vi "dummy.vi"() -> ()   [LabVIEW 2021]
panel:
  in  "stop":bool
  in  "RPM":dbl(slide) scale=1.0..500.0
  out "Visualize":bool[](array[boolean])
  in  "Full Step":bool
  in  "Direction":enum32{"CW", "CCW"}(radio)
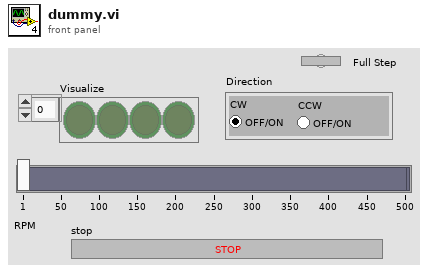
[diagram p1: front panel]
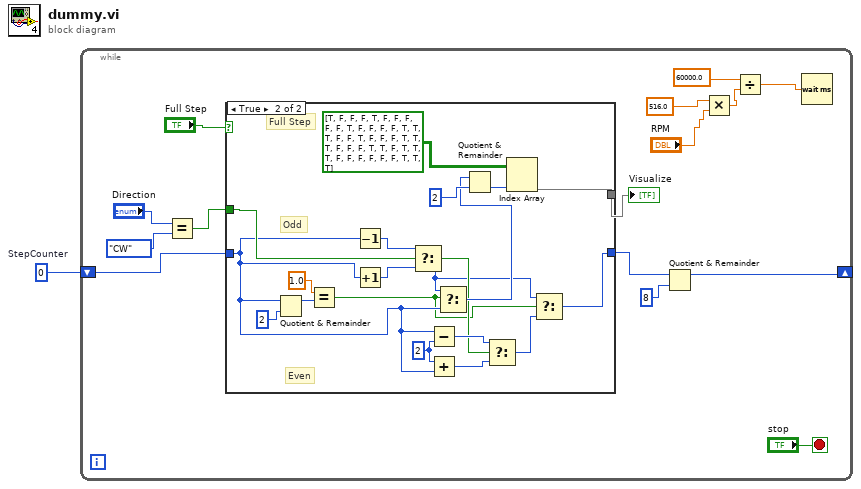
[diagram p0: block diagram]
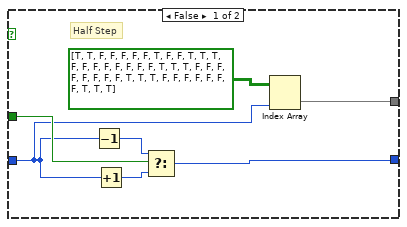
[diagram p2: hidden frame]
diagram:
  w1 = 0  # StepCounter
  n1 = while {
    shift-right: [w11] -> _
    shift-left: w1 -> [w14]
    stop <- "stop" stop-if-true
    n2 = Equal?(x="Direction", y=enum32{"CW", "CCW"}."CW") -> (x = y?=w8:bool)
    n3 = case shown="True" "Full Step" {
      tunnel: w14 -> [w17 w28]
      tunnel: [w19 w24] -> w13
      tunnel: w8 -> [w23 w30]
      tunnel: [w22 w32] -> w7
      frame False {
        # "Half Step"
        n4 = Decrement(x=w17) -> (x-1=w21:i32)
        n5 = Increment(x=w17) -> (x+1=w20:i32)
        n6 = Select(t=w21, s=w23, f=w20) -> (s? t:f=w19:i32)
        n7 = Index Array(array=bool[][] [[TRUE, TRUE, FALSE, FALSE, FALSE, FALSE, FALSE, TRUE, FALSE], [FALSE, TRUE, TRUE, TRUE, FALSE, FALSE, FALSE, FALSE, FALSE], [FALSE, FALSE, FALSE, TRUE, TRUE, TRUE, FALSE, FALSE, FALSE], [FALSE, FALSE, FALSE, FALSE, FALSE, TRUE, TRUE, TRUE, FALSE], [FALSE, FALSE, FALSE, FALSE, FALSE, FALSE, TRUE, TRUE, TRUE]], index (col)=w17) -> (element=w22:bool[])  [unwired: 1 in]
      }
      frame True {
        w42 = 2 ("y")
        # "Odd"
        # "Even"
        # "Full Step"
        n8 = Quotient & Remainder(x=w28, y=2) -> (x-y*floor(x/y)=w38:i32)  [unwired: 1 out]
        n9 = Equal?(x=1.0, y=w38) -> (x = y?=w27:bool)
        n10 = Decrement(x=w28) -> (x-1=w37:i32)
        n11 = Increment(x=w28) -> (x+1=w36:i32)
        n12 = Select(t=w37, s=w30, f=w36) -> (s? t:f=w26:i32)
        n13 = Subtract(x=w28, y=w42) -> (x-y=w41:i32)
        n14 = Add(x=w42, y=w28) -> (x+y=w35:i32)
        n15 = Select(t=w26, s=w27, f=w28) -> (s? t:f=w31:i32)
        n16 = Quotient & Remainder(x=w31, y=2) -> (floor(x/y)=w29:i32)  [unwired: 1 out]
        n17 = Select(t=w41, s=w30, f=w35) -> (s? t:f=w25:i32)
        n18 = Index Array(array=bool[][] [[TRUE, FALSE, FALSE, FALSE, TRUE, FALSE, FALSE, FALSE, FALSE], [FALSE, TRUE, FALSE, FALSE, FALSE, FALSE, TRUE, TRUE, TRUE], [FALSE, FALSE, TRUE, FALSE, FALSE, FALSE, TRUE, TRUE, TRUE], [FALSE, FALSE, FALSE, TRUE, TRUE, FALSE, TRUE, TRUE, TRUE], [FALSE, FALSE, FALSE, FALSE, FALSE, FALSE, TRUE, TRUE, TRUE]], index (col)=w29) -> (element=w32:bool[])  [unwired: 1 in]
        n19 = Select(t=w26, s=w27, f=w25) -> (s? t:f=w24:i32)
      }
    }
    "Visualize" <- w7
    n20 = Quotient & Remainder(x=w13, y=8) -> (x-y*floor(x/y)=w11:i32)  [unwired: 1 out]
    n21 = Multiply(x=516.0 ("y"), y="RPM") -> (x*y=w3:dbl)
    n22 = Divide(x=60000.0 ("y"), y=w3) -> (x/y=w2:dbl)
    n23 = Wait (ms)(milliseconds to wait=w2) -> ()  [unwired: 1 out]
  }
